vi "停止整机测试(子VI).vi"() -> (0 "error out":T1={"status"=FALSE, "代码"=4, "source"=""} caption="错误输出" {"代码" items=["执行成功"=1, "执行失败，但不知道原因"=2, "命令请求条件错误"=3, "通讯超时"=4, "系统繁忙不能执行"=5, "系统故障"=6, "没有数据"=100]})   [LabVIEW 2016, in "MB SLAVE.lvlib"]
uses:
  MB SLAVE.lvlib
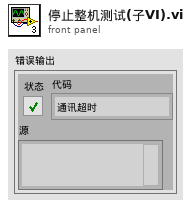
[diagram p1: front panel]
types:
  T1 = cluster{"status":bool, "代码":u16, "source":string}
  T2 = cluster{"命令":string, cluster{"starting address":u16, "holding register value":u16}}
  T3 = cluster{"命令":string, "测量模式":enum16{"水样测量", "标样核查", "零点核查", "跨度核查", "空白测试", "加标回收", "平行样", "校零", "校标"}, "CODMn量程切换":enum32{"H", "L", "AUTO"}}
  T4 = typedef "启动参数.ctl" = cluster{"氨氮":bool, "总磷":bool, "总氮":bool, "多参数":bool, "CODmn":bool, "CODCr":bool, "氟化物":bool, "超标留样启用":bool, "重金属":bool}
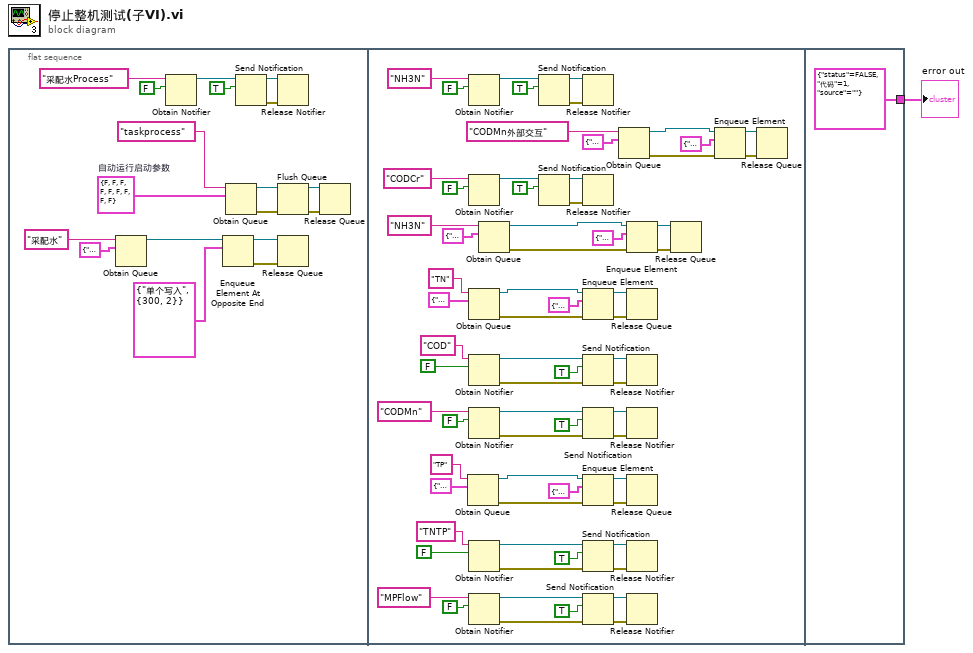
[diagram p0: block diagram]
diagram:
  n1 = flat-sequence {
    tunnel: [T1 {"status"=FALSE, "代码"=1, "source"=""} ("error out")] -> w1
    frame #0 {
      w2 = T4 {"氨氮"=FALSE, "总磷"=FALSE, "总氮"=FALSE, "多参数"=FALSE, "CODmn"=FALSE, "CODCr"=FALSE, "氟化物"=FALSE, "超标留样启用"=FALSE, "重金属"=FALSE}  # 自动运行启动参数
      n2 = Obtain Queue(name (unnamed)="采配水" ("名称（未命名）"), element data type=cluster{"命令":string, "数据":variant} {"命令"="", "数据"=variant}) -> (queue out=w17:refnum<queue>)  [unwired: 3 in, 2 out]
      n3 = Obtain Notifier(name (unnamed)="采配水Process" ("名称（未命名）"), notification data type=FALSE) -> (notifier out=w19:refnum<notifier>)  [unwired: 2 in, 2 out]
      n4 = Enqueue Element At Opposite End(queue=w17, element=T2 {"命令"="单个写入", {"starting address"=300, "holding register value"=2}} ("元素")) -> (queue out=w11:refnum<queue>, error out=w10:errorcluster)  [unwired: 2 in, 1 out]
      n5 = Obtain Queue(name (unnamed)="taskprocess" ("名称（未命名）"), element data type=w2) -> (queue out=w6:refnum<queue>, error out=w5:errorcluster)  [unwired: 3 in, 1 out]
      n6 = Send Notification(notification=TRUE ("通知"), notifier=w19) -> (notifier out=w9:refnum<notifier>, error out=w8:errorcluster)  [unwired: 1 in]
      n7 = Release Notifier(notifier=w9, error in (no error)=w8) -> ()  [unwired: 1 in, 3 out]
      n8 = Flush Queue(queue=w6, error in (no error)=w5) -> (queue out=w3:refnum<queue>, error out=w4:errorcluster)  [unwired: 1 out]
      n9 = Release Queue(queue=w11, error in (no error)=w10) -> ()  [unwired: 1 in, 3 out]
      n10 = Release Queue(queue=w3, error in (no error)=w4) -> ()  [unwired: 1 in, 3 out]
    }
    frame #1 {
      n11 = Obtain Queue(name (unnamed)="TP" ("名称（未命名）"), element data type=cluster{"命令":string, "data":variant} {"命令"="", "data"=variant}) -> (queue out=w80:refnum<queue>, error out=w57:errorcluster)  [unwired: 3 in, 1 out]
      n12 = Obtain Notifier(name (unnamed)="NH3N" ("名称（未命名）"), notification data type=FALSE) -> (notifier out=w84:refnum<notifier>)  [unwired: 2 in, 2 out]
      n13 = Obtain Notifier(name (unnamed)="CODCr" ("名称（未命名）"), notification data type=FALSE) -> (notifier out=w63:refnum<notifier>)  [unwired: 2 in, 2 out]
      n14 = Obtain Queue(name (unnamed)="TN" ("名称（未命名）"), element data type=cluster{"命令":string, "data":variant} {"命令"="", "data"=variant}) -> (queue out=w53:refnum<queue>, error out=w52:errorcluster)  [unwired: 3 in, 1 out]
      n15 = Obtain Notifier(name (unnamed)="COD" ("名称（未命名）"), notification data type=FALSE) -> (notifier out=w32:refnum<notifier>, error out=w33:errorcluster)  [unwired: 2 in, 1 out]
      n16 = Obtain Notifier(name (unnamed)="CODMn" ("名称（未命名）"), notification data type=FALSE) -> (notifier out=w69:refnum<notifier>, error out=w28:errorcluster)  [unwired: 2 in, 1 out]
      n17 = Obtain Notifier(name (unnamed)="TNTP" ("名称（未命名）"), notification data type=FALSE) -> (notifier out=w76:refnum<notifier>, error out=w27:errorcluster)  [unwired: 2 in, 1 out]
      n18 = Obtain Notifier(name (unnamed)="MPFlow" ("名称（未命名）"), notification data type=FALSE) -> (notifier out=w65:refnum<notifier>, error out=w64:errorcluster)  [unwired: 2 in, 1 out]
      n19 = Obtain Queue(name (unnamed)="NH3N" ("名称（未命名）"), element data type=cluster{"命令":string, "data":variant} {"命令"="", "data"=variant}) -> (queue out=w87:refnum<queue>, error out=w56:errorcluster)  [unwired: 3 in, 1 out]
      n20 = Send Notification(notification=TRUE ("通知"), notifier=w84) -> (notifier out=w45:refnum<notifier>, error out=w44:errorcluster)  [unwired: 1 in]
      n21 = Send Notification(notification=TRUE ("通知"), notifier=w63) -> (notifier out=w39:refnum<notifier>, error out=w38:errorcluster)  [unwired: 1 in]
      n22 = Release Notifier(notifier=w45, error in (no error)=w44) -> ()  [unwired: 1 in, 3 out]
      n23 = Release Notifier(notifier=w39, error in (no error)=w38) -> ()  [unwired: 1 in, 3 out]
      n24 = Enqueue Element(queue=w53, element=cluster{"命令":string, "data":variant} {"命令"="启动", "data"=variant(cluster{"站号":u16, "控制命令输出":u16[]} {"站号"=2, "控制命令输出"=[2816]})} ("元素"), error in (no error)=w52) -> (queue out=w51:refnum<queue>, error out=w50:errorcluster)  [unwired: 1 in, 1 out]
      n25 = Send Notification(notification=TRUE ("通知"), notifier=w32, error in (no error)=w33) -> (notifier out=w34:refnum<notifier>, error out=w35:errorcluster)
      n26 = Send Notification(notification=TRUE ("通知"), notifier=w69, error in (no error)=w28) -> (notifier out=w41:refnum<notifier>, error out=w40:errorcluster)
      n27 = Enqueue Element(queue=w80, element=cluster{"命令":string, "data":variant} {"命令"="启动", "data"=variant(cluster{"站号":u16, "控制命令输出":u16[]} {"站号"=1, "控制命令输出"=[2816]})} ("元素"), error in (no error)=w57) -> (queue out=w49:refnum<queue>, error out=w48:errorcluster)  [unwired: 1 in, 1 out]
      n28 = Send Notification(notification=TRUE ("通知"), notifier=w76, error in (no error)=w27) -> (notifier out=w43:refnum<notifier>, error out=w42:errorcluster)
      n29 = Send Notification(notification=TRUE ("通知"), notifier=w65, error in (no error)=w64) -> (notifier out=w37:refnum<notifier>, error out=w36:errorcluster)
      n30 = Obtain Queue(name (unnamed)="CODMn外部交互" ("名称（未命名）"), element data type=T3 {"命令"="启动命令", "测量模式"=enum."水样测量", "CODMn量程切换"=enum."AUTO"} ("元素")) -> (queue out=w22:refnum<queue>, error out=w21:errorcluster)  [unwired: 3 in, 1 out]
      n31 = Enqueue Element(queue=w87, element=cluster{"命令":string, "data":variant} {"命令"="启动", "data"=variant(cluster{"站号":u16, "控制命令输出":u16[]} {"站号"=3, "控制命令输出"=[2816]})} ("启动命令"), error in (no error)=w56) -> (queue out=w47:refnum<queue>, error out=w46:errorcluster)  [unwired: 1 in, 1 out]
      n32 = Release Queue(queue=w51, error in (no error)=w50) -> ()  [unwired: 1 in, 3 out]
      n33 = Release Notifier(notifier=w34, error in (no error)=w35) -> ()  [unwired: 1 in, 3 out]
      n34 = Release Notifier(notifier=w41, error in (no error)=w40) -> ()  [unwired: 1 in, 3 out]
      n35 = Release Queue(queue=w49, error in (no error)=w48) -> ()  [unwired: 1 in, 3 out]
      n36 = Release Notifier(notifier=w43, error in (no error)=w42) -> ()  [unwired: 1 in, 3 out]
      n37 = Release Notifier(notifier=w37, error in (no error)=w36) -> ()  [unwired: 1 in, 3 out]
      n38 = Release Queue(queue=w47, error in (no error)=w46) -> ()  [unwired: 1 in, 3 out]
      n39 = Enqueue Element(queue=w22, element=T3 {"命令"="停止命令", "测量模式"=enum."水样测量", "CODMn量程切换"=enum."H"} ("元素"), error in (no error)=w21) -> (queue out=w24:refnum<queue>, error out=w23:errorcluster)  [unwired: 1 in, 1 out]
      n40 = Release Queue(queue=w24, error in (no error)=w23) -> ()  [unwired: 1 in, 3 out]
    }
    frame #2 {
    }
  }
  "error out" <- w1
